vi "Display Dialog.vi"(8 "error in (no error)":errorcluster, 10 "Argument":string, 11 "State Data":T1={"Core"={"Current VI Reference"=refnum, "Close Panel on Exit?"=FALSE}, "FP Refs"={"VI Tree"=refnum, "Window Title"=refnum, "Same Title as VI?"=refnum, "VI Desc"=refnum, "Help Path"=refnum, "Help Tag"=refnum, "Help URL"=refnum, "Help Type"=refnum, "Controls"=refnum, "VI Connector Pane"=refnum, "Path to VI"=refnum, "Inlined?"=refnum, "Allow Debugging?"=refnum, "Auto Error Handling?"=refnum, "Run When Opened?"=refnum, "Suspend When Called?"=refnum, "Reentrancy"=refnum, "Priority"=refnum, "Preferred Exec System"=refnum, "VI Type"=refnum, "Help Properties"=refnum, "Edit Icon"=refnum, "Add Copyright"=refnum, "Set all VIs"=refnum}, "Current Path"=path "", "New Item Data"=[], "Saved Item Data"=[], "FP"={"Selected VI Data"=0, "Help Path"="", "Help Tag"="", "Help URL"="", "Help Type"=enum."Local Help File", "VI Desc"="", "Controls"=[], "Window Title"="", "Same Title?"=FALSE, "VI Tree Value"=""}, "Config Path"=path "", "Config"={"ItemsEdited"=0, "Copyright Path"=path "", "Copyright Delimiter"="", "Recent Folders"=[], "Recent Files"=[], "Recent Filters"=[], "Abbreviate Names?"=FALSE, "Format Bold Tags?"=FALSE, "Show ConPane Only?"=FALSE, "Show Top-Level Only?"=FALSE, "Confirm Save?"=FALSE, "Confirm Revert?"=FALSE, "Confirm Save All?"=FALSE, "Confirm Revert All?"=FALSE, "Confirm Exit?"=FALSE, "Flat View?"=FALSE, "Ctls Sort Column"=0, "Ctls Sort Order"=0}, "Desc Selection"={"Selection Start"=0, "Selection End"=0}, "Displayed Indices"=[], "Filter"={"Filter Column"=enum."Description", "Filter Type"=enum."Contains", "Filter Value"="", "New Data?"=FALSE, "Case Sensitive?"=FALSE, "Enabled?"=FALSE}, "Sort"={"Sort Column"=enum."Description", "Ascending?"=FALSE, "Enabled?"=FALSE}, "Tree Map"=refnum, "Last Save Count"=0, "View Saved?"=FALSE, "Selected Item"=refnum}) -> (0 "error out":errorcluster, 1 "States at Back":string, 2 "States at Front":string, 3 "State Data out":T1={"Core"={"Current VI Reference"=refnum, "Close Panel on Exit?"=FALSE}, "FP Refs"={"VI Tree"=refnum, "Window Title"=refnum, "Same Title as VI?"=refnum, "VI Desc"=refnum, "Help Path"=refnum, "Help Tag"=refnum, "Help URL"=refnum, "Help Type"=refnum, "Controls"=refnum, "VI Connector Pane"=refnum, "Path to VI"=refnum, "Inlined?"=refnum, "Allow Debugging?"=refnum, "Auto Error Handling?"=refnum, "Run When Opened?"=refnum, "Suspend When Called?"=refnum, "Reentrancy"=refnum, "Priority"=refnum, "Preferred Exec System"=refnum, "VI Type"=refnum, "Help Properties"=refnum, "Edit Icon"=refnum, "Add Copyright"=refnum, "Set all VIs"=refnum}, "Current Path"=path "", "New Item Data"=[], "Saved Item Data"=[], "FP"={"Selected VI Data"=0, "Help Path"="", "Help Tag"="", "Help URL"="", "Help Type"=enum."Local Help File", "VI Desc"="", "Controls"=[], "Window Title"="", "Same Title?"=FALSE, "VI Tree Value"=""}, "Config Path"=path "", "Config"={"ItemsEdited"=0, "Copyright Path"=path "", "Copyright Delimiter"="", "Recent Folders"=[], "Recent Files"=[], "Recent Filters"=[], "Abbreviate Names?"=FALSE, "Format Bold Tags?"=FALSE, "Show ConPane Only?"=FALSE, "Show Top-Level Only?"=FALSE, "Confirm Save?"=FALSE, "Confirm Revert?"=FALSE, "Confirm Save All?"=FALSE, "Confirm Revert All?"=FALSE, "Confirm Exit?"=FALSE, "Flat View?"=FALSE, "Ctls Sort Column"=0, "Ctls Sort Order"=0}, "Desc Selection"={"Selection Start"=0, "Selection End"=0}, "Displayed Indices"=[], "Filter"={"Filter Column"=enum."Description", "Filter Type"=enum."Contains", "Filter Value"="", "New Data?"=FALSE, "Case Sensitive?"=FALSE, "Enabled?"=FALSE}, "Sort"={"Sort Column"=enum."Description", "Ascending?"=FALSE, "Enabled?"=FALSE}, "Tree Map"=refnum, "Last Save Count"=0, "View Saved?"=FALSE, "Selected Item"=refnum})   [LabVIEW 2020, in "VI Properties Editor.lvlib"]
doc: "Displays an appropriate dialog according to <B>Argument</B>, and outputs any states that should be enqueued after the dialog is closed."
uses:
  VI Properties Editor.lvlib
  CTLs/Main State Data.ctl
  Classes/Tree Map/Project Tree Map.lvclass
  Classes/Item/Item.lvclass
  CTLs/Main References.ctl
  CTLs/Main Front Panel Controls.ctl
  CTLs/Config.ctl
  CTLs/Filter Info.ctl
  CTLs/Filter Column.ctl
  CTLs/Filter Type.ctl
  <vilib>/Utility/miscctls.llb/LVSelectionTypeDef.ctl
  CTLs/Sort Info.ctl
  CTLs/Sort Column.ctl
  CTLs/Confirmation Type.ctl
  <vilib>/LabVIEW Icon API/lv_icon/Classes/Icon/Icon.lvclass
  <vilib>/LabVIEW Icon API/LabVIEW Icon API.lvlib
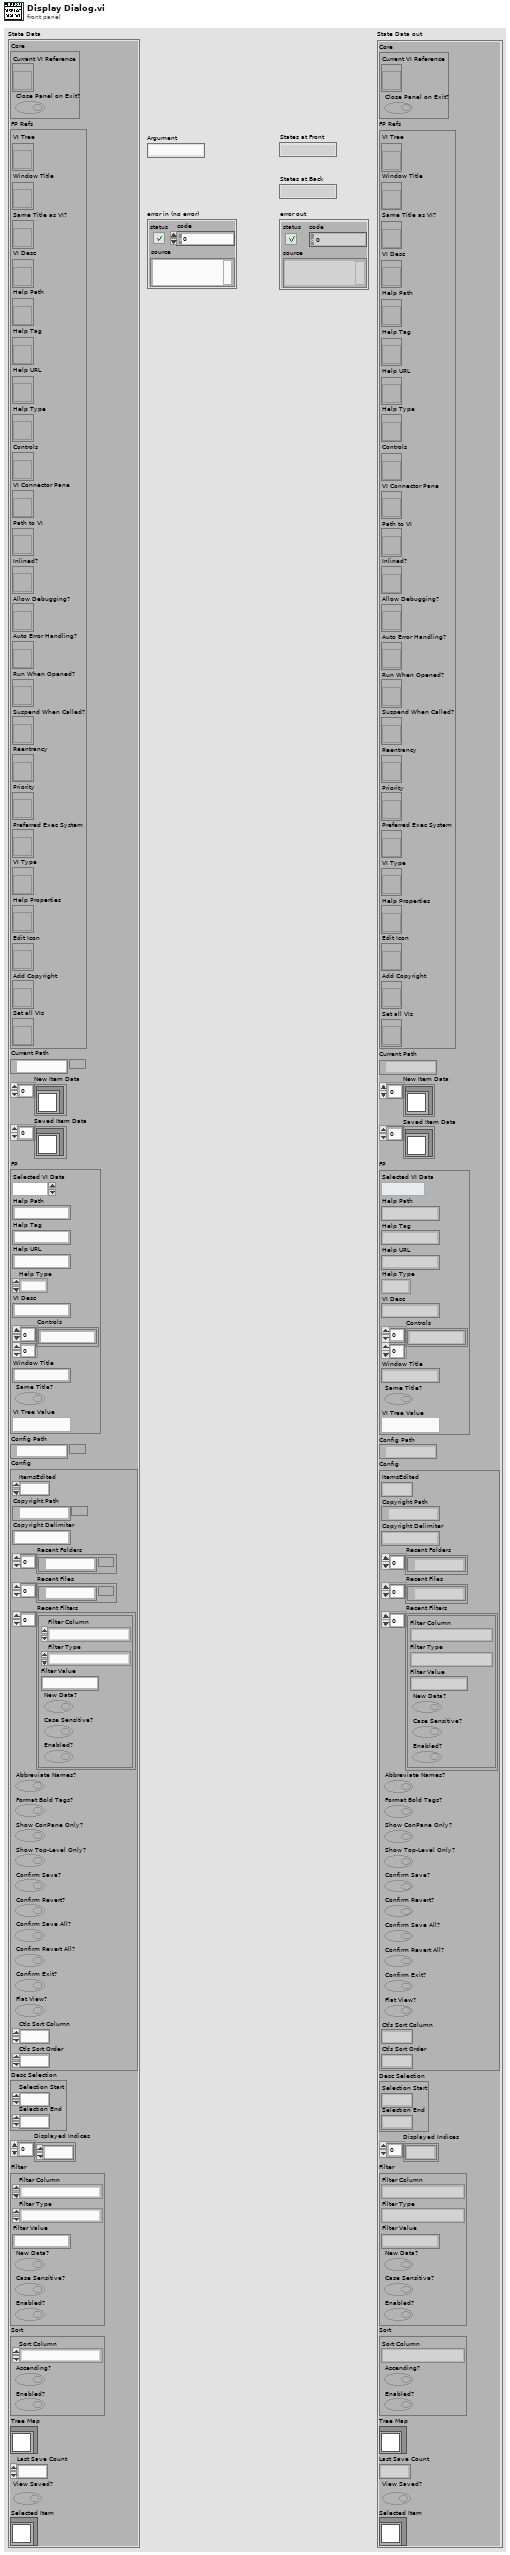
[diagram p1: front panel]
types:
  T1 = typedef "VI Properties Editor.lvlib/Main State Data.ctl" = cluster{"Core":cluster{"Current VI Reference":refnum<vi>, "Close Panel on Exit?":bool}, "FP Refs":T2, "Current Path":path, "New Item Data":refnum<class "Item.lvclass">[], "Saved Item Data":refnum<class "Item.lvclass">[], "FP":T3, "Config Path":path, "Config":T4, "Desc Selection":T8, "Displayed Indices":i32[], "Filter":T5, "Sort":T9, "Tree Map":refnum<class "Project Tree Map.lvclass">, "Last Save Count":u32, "View Saved?":bool, "Selected Item":refnum<class "Item.lvclass">}
  T2 = typedef "VI Properties Editor.lvlib/Main References.ctl" = cluster{"VI Tree":refnum<vi>, "Window Title":refnum<vi>, "Same Title as VI?":refnum<vi>, "VI Desc":refnum<vi>, "Help Path":refnum<vi>, "Help Tag":refnum<vi>, "Help URL":refnum<vi>, "Help Type":refnum<vi>, "Controls":refnum<vi>, "VI Connector Pane":refnum<vi>, "Path to VI":refnum<vi>, "Inlined?":refnum<vi>, "Allow Debugging?":refnum<vi>, "Auto Error Handling?":refnum<vi>, "Run When Opened?":refnum<vi>, "Suspend When Called?":refnum<vi>, "Reentrancy":refnum<vi>, "Priority":refnum<vi>, "Preferred Exec System":refnum<vi>, "VI Type":refnum<vi>, "Help Properties":refnum<vi>, "Edit Icon":refnum<vi>, "Add Copyright":refnum<vi>, "Set all VIs":refnum<vi>}
  T3 = typedef "VI Properties Editor.lvlib/Main Front Panel Controls.ctl" = cluster{"Selected VI Data":i32, "Help Path":string, "Help Tag":string, "Help URL":string, "Help Type":enum16{"Local Help File", "Web-based Help"}, "VI Desc":string, "Controls":string[][], "Window Title":string, "Same Title?":bool, "VI Tree Value":string}
  T4 = typedef "VI Properties Editor.lvlib/Config.ctl" = cluster{"ItemsEdited":u32, "Copyright Path":path, "Copyright Delimiter":string, "Recent Folders":path[], "Recent Files":path[], "Recent Filters":T5[], "Abbreviate Names?":bool, "Format Bold Tags?":bool, "Show ConPane Only?":bool, "Show Top-Level Only?":bool, "Confirm Save?":bool, "Confirm Revert?":bool, "Confirm Save All?":bool, "Confirm Revert All?":bool, "Confirm Exit?":bool, "Flat View?":bool, "Ctls Sort Column":i32, "Ctls Sort Order":i32}
  T5 = typedef "VI Properties Editor.lvlib/Filter Info.ctl" = cluster{"Filter Column":T6, "Filter Type":T7, "Filter Value":string, "New Data?":bool, "Case Sensitive?":bool, "Enabled?":bool}
  T6 = typedef "VI Properties Editor.lvlib/Filter Column.ctl" = enum16{"Name", "Path", "Type", "Window Title", "Description", "Help Path", "Help Tag", "Custom Title?", "Reentrancy", "Inlined?", "Help URL", "Help Type", "Allow Debugging?", "Auto Error Handling?", "Run When Opened?", "Suspend When Called?", "Priority", "Preferred Exec Sytem", "Control Label", "Control Caption", "Control Description", "Control Tip Strip"}
  T7 = typedef "VI Properties Editor.lvlib/Filter Type.ctl" = enum16{"Contains", "Equals", "Starts with", "Ends with", "Is empty", "Does not contain", "Does not equal", "Is not empty"}
  T8 = typedef "LVSelectionTypeDef.ctl" = cluster{"Selection Start":u32, "Selection End":u32}
  T9 = typedef "VI Properties Editor.lvlib/Sort Info.ctl" = cluster{"Sort Column":T10, "Ascending?":bool, "Enabled?":bool}
  T10 = typedef "VI Properties Editor.lvlib/Sort Column.ctl" = enum16{"Name", "Filename", "Path", "Type", "Window Title", "Description", "Help Path", "Help Tag", "Custom Title?", "Reentrancy", "Inlined?", "Help URL", "Help Type", "Allow Debugging?", "Auto Error Handling?", "Run When Opened?", "Suspend When Called?", "Priority", "Preferred Exec Sytem"}
  T11 = enum16{"Left Button", "Center Button", "Right Button", "Window Close"}
  T12 = typedef "VI Properties Editor.lvlib/Confirmation Type.ctl" = enum16{"Save", "Revert", "Save All", "Revert All", "Exit"}
  T13 = typedef "VI Properties Editor.lvlib/Replace Info.ctl" = cluster{"Filter Column":T6, "Filter Type":T7, "Filter Value":string, "Case Sensitive?":bool, "Replace Column":T14, "Replace Value":string}
  T14 = typedef "VI Properties Editor.lvlib/Replace Column.ctl" = enum16{"Window Title", "Description", "Help Path", "Help Tag", "Custom Title?", "Help URL", "Help Type", "Control Label", "Control Caption", "Control Description", "Control Tip Strip"}
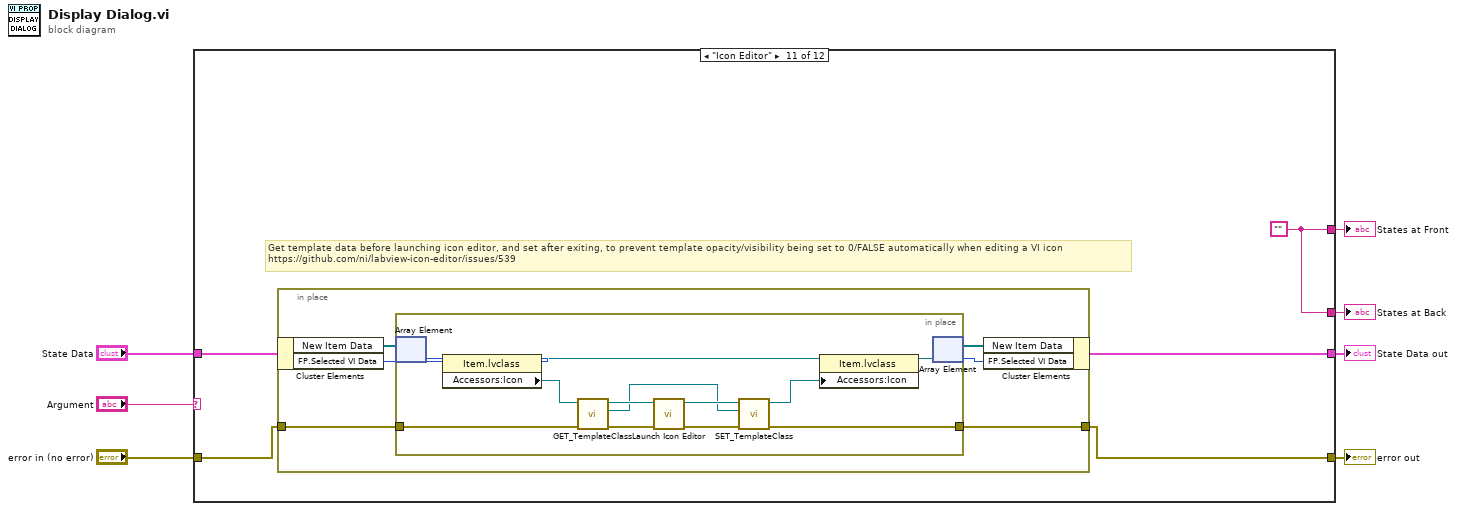
[diagram p0: block diagram]
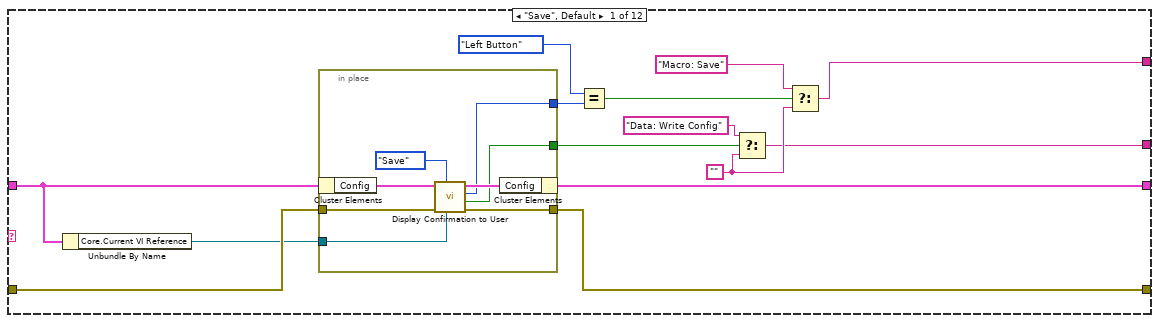
[diagram p2: hidden frame]
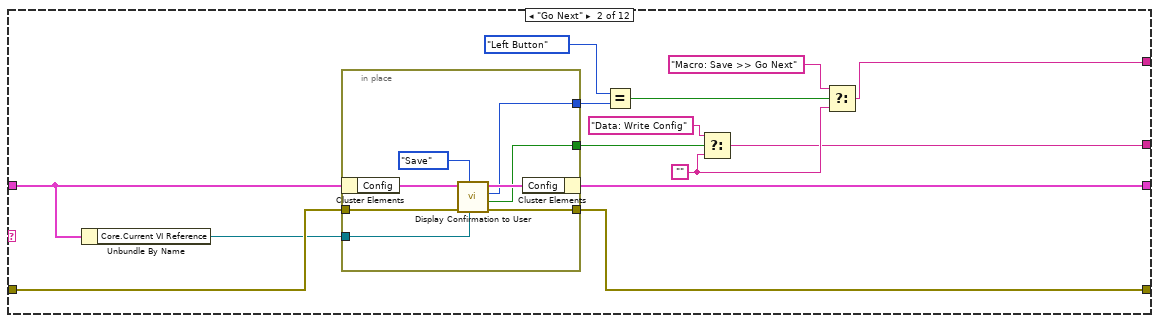
[diagram p3: hidden frame]
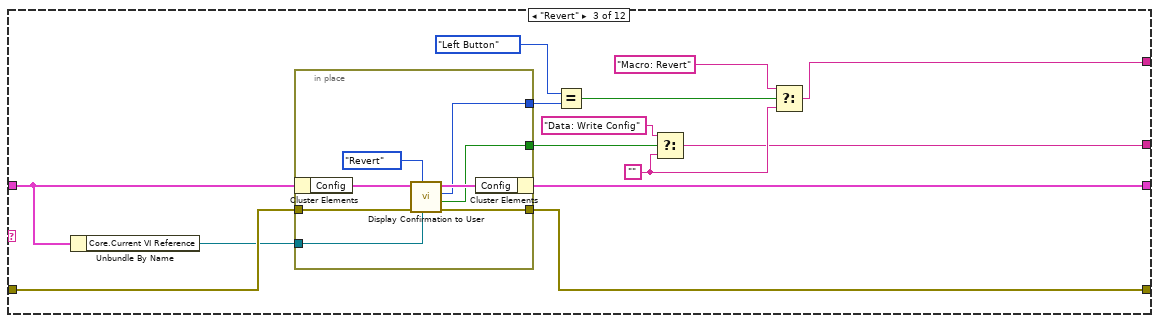
[diagram p4: hidden frame]
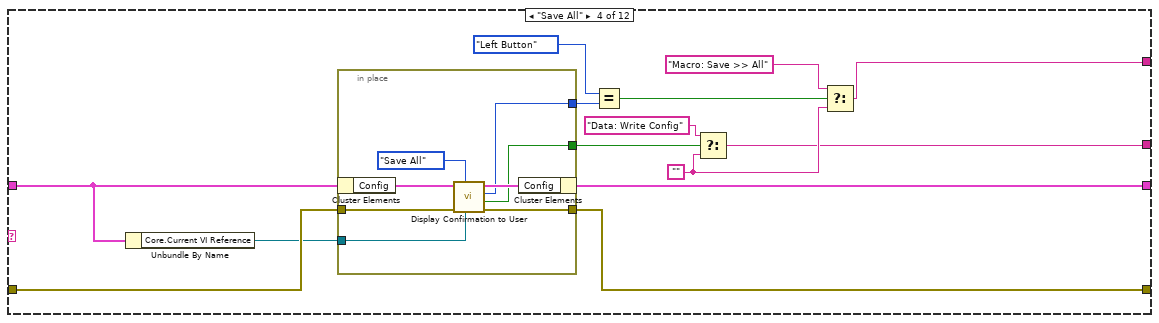
[diagram p5: hidden frame]
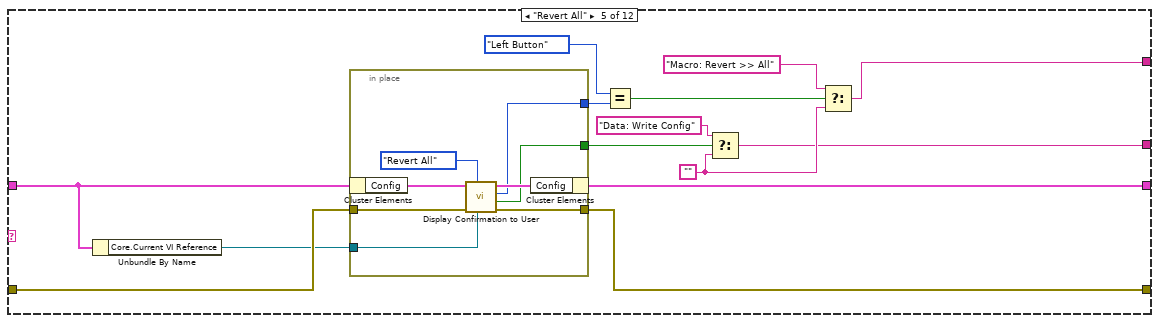
[diagram p6: hidden frame]
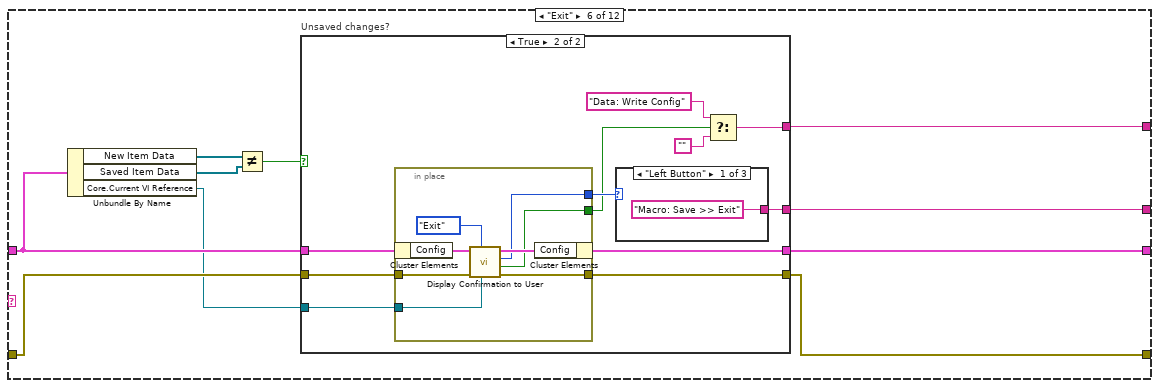
[diagram p7: hidden frame]
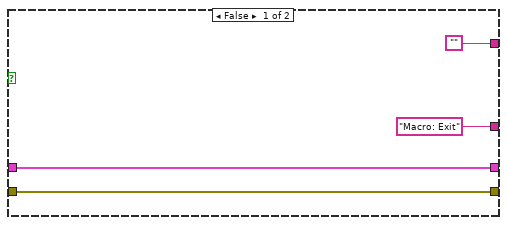
[diagram p8: hidden frame]
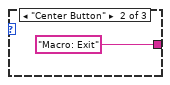
[diagram p9: hidden frame]
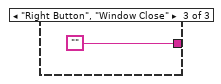
[diagram p10: hidden frame]
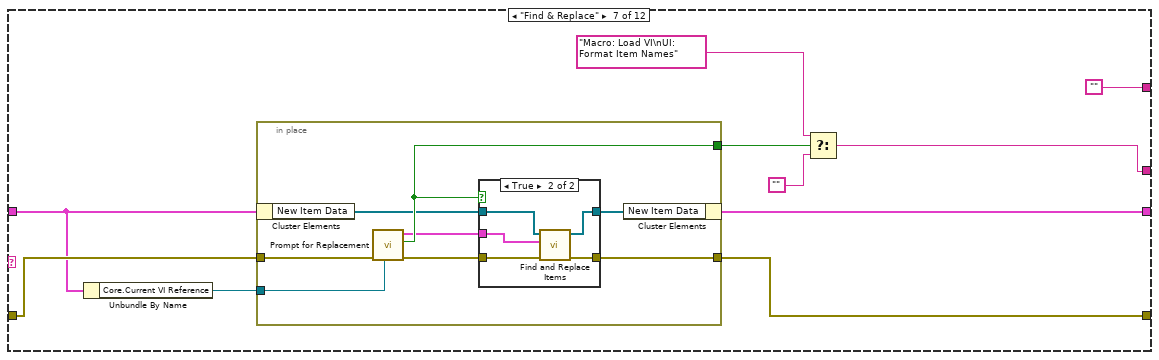
[diagram p11: hidden frame]
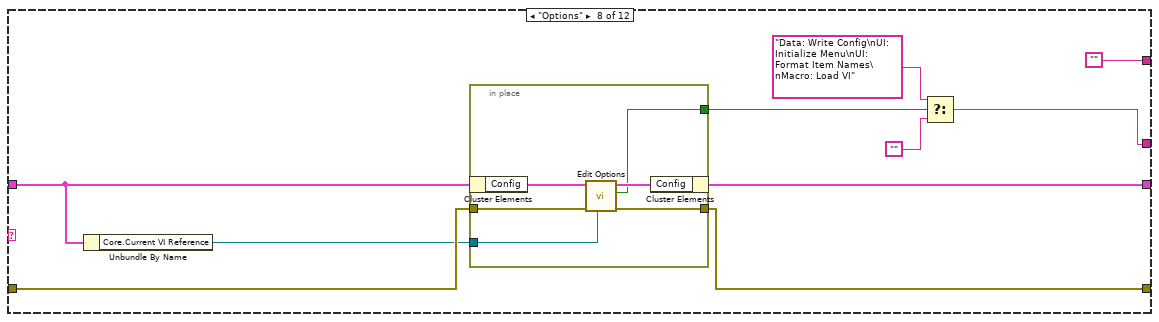
[diagram p13: hidden frame]
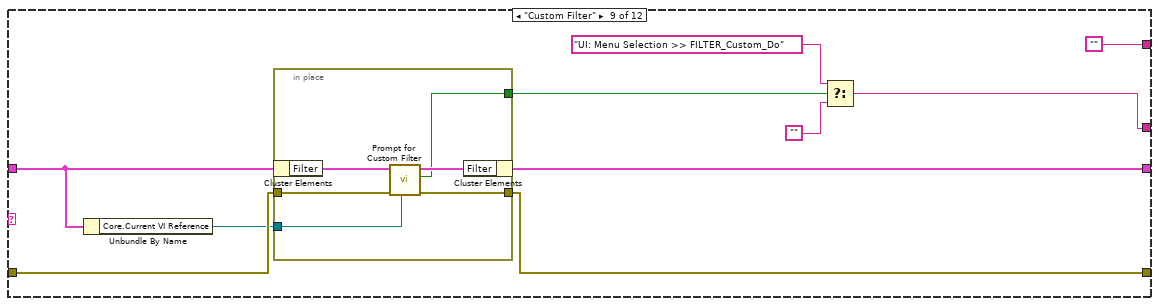
[diagram p14: hidden frame]
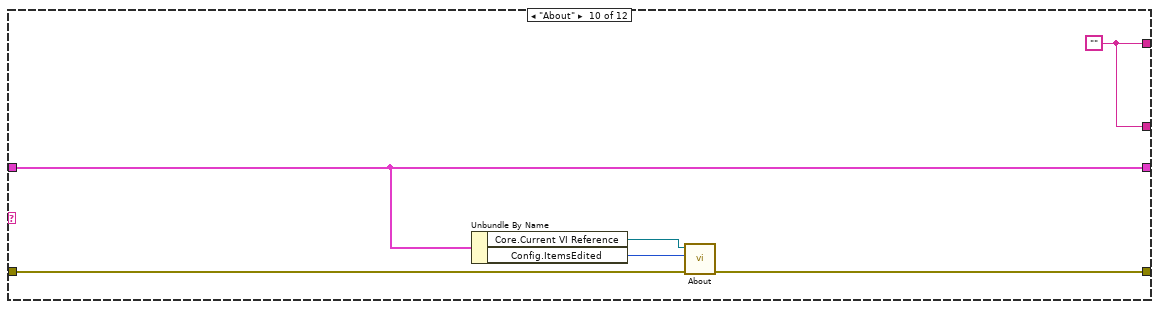
[diagram p15: hidden frame]
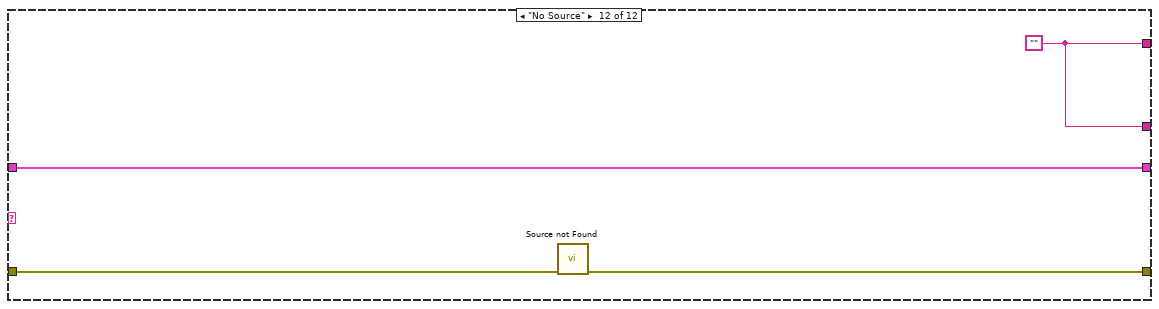
[diagram p16: hidden frame]
diagram:
  n1 = case shown="\"Icon Editor\"" "Argument" {
    tunnel: [w13 w35 w58 w80 w102 w125 "" "" "" w216 w221 w243] -> w2
    tunnel: "error in (no error)" -> [w21 w43 w65 w87 w109 w122 w160 w183 w199 w214 w220 w241]
    tunnel: "State Data" -> [w9 w31 w53 w75 w97 w123 w159 w184 w200 w212 w217 w242]
    tunnel: [w20 w42 w64 w86 w108 w121 w157 w181 w198 w213 w219 w240] -> w4
    tunnel: [w19 w41 w63 w85 w107 w120 w156 w182 w195 w212 w218 w242] -> w6
    tunnel: [w14 w36 w57 w79 w101 w119 w155 w180 w196 w216 w221 w243] -> w3
    frame "Save", Default {
      w16 = ""
      n2 = Unbundle By Name(w9) -> ("Core.Current VI Reference"=w8:refnum<vi>)
      n3 = in-place {
        in-place-border: w21 -> [w28]
        in-place-border: [w26] -> w20
        in-place-border: [w24] -> w18
        in-place-border: [w23] -> w11
        in-place-border: w8 -> [w22]
        n4 = in-place-cluster #1(w9) -> ("Config"=w29:T4)
        n5 = call "Display Confirmation to User.vi"("Calling VI in"=w22, "Confirmation Type"=Confirmation_Type."Save", "error in (no error)"=w28, "Config"=w29) -> ("error out"=w26:errorcluster, "New Config?"=w24:bool, "Which Button?"=w23:T11, "Config out"=w27:T4)  [unwired: 4 in]
        n6 = in-place-cluster #1("Config"=w27) -> (w19:T1)
      }
      n7 = Equal?(x=T11."Left Button", y=w11) -> (x = y?=w10:bool)
      n8 = Select(t="Data: Write Config", s=w18, f=w16) -> (s? t:f=w14:string)
      n9 = Select(t="Macro: Save", s=w10, f=w16) -> (s? t:f=w13:string)
    }
    frame "Go Next" {
      w38 = ""
      n10 = Unbundle By Name(w31) -> ("Core.Current VI Reference"=w30:refnum<vi>)
      n11 = in-place {
        in-place-border: w43 -> [w50]
        in-place-border: [w48] -> w42
        in-place-border: [w46] -> w40
        in-place-border: [w45] -> w33
        in-place-border: w30 -> [w44]
        n12 = in-place-cluster #2(w31) -> ("Config"=w51:T4)
        n13 = call "Display Confirmation to User.vi"("Calling VI in"=w44, "Confirmation Type"=Confirmation_Type."Save", "error in (no error)"=w50, "Config"=w51) -> ("error out"=w48:errorcluster, "New Config?"=w46:bool, "Which Button?"=w45:T11, "Config out"=w49:T4)  [unwired: 4 in]
        n14 = in-place-cluster #2("Config"=w49) -> (w41:T1)
      }
      n15 = Equal?(x=T11."Left Button", y=w33) -> (x = y?=w32:bool)
      n16 = Select(t="Data: Write Config", s=w40, f=w38) -> (s? t:f=w36:string)
      n17 = Select(t="Macro: Save >> Go Next", s=w32, f=w38) -> (s? t:f=w35:string)
    }
    frame "Revert" {
      w60 = ""
      n18 = Unbundle By Name(w53) -> ("Core.Current VI Reference"=w52:refnum<vi>)
      n19 = in-place {
        in-place-border: w65 -> [w72]
        in-place-border: [w70] -> w64
        in-place-border: [w68] -> w62
        in-place-border: [w67] -> w55
        in-place-border: w52 -> [w66]
        n20 = in-place-cluster #3(w53) -> ("Config"=w73:T4)
        n21 = call "Display Confirmation to User.vi"("Calling VI in"=w66, "Confirmation Type"=Confirmation_Type."Revert", "error in (no error)"=w72, "Config"=w73) -> ("error out"=w70:errorcluster, "New Config?"=w68:bool, "Which Button?"=w67:T11, "Config out"=w71:T4)  [unwired: 4 in]
        n22 = in-place-cluster #3("Config"=w71) -> (w63:T1)
      }
      n23 = Equal?(x=T11."Left Button", y=w55) -> (x = y?=w54:bool)
      n24 = Select(t="Data: Write Config", s=w62, f=w60) -> (s? t:f=w57:string)
      n25 = Select(t="Macro: Revert", s=w54, f=w60) -> (s? t:f=w58:string)
    }
    frame "Save All" {
      w82 = ""
      n26 = Unbundle By Name(w75) -> ("Core.Current VI Reference"=w74:refnum<vi>)
      n27 = in-place {
        in-place-border: w87 -> [w94]
        in-place-border: [w92] -> w86
        in-place-border: [w90] -> w84
        in-place-border: [w89] -> w77
        in-place-border: w74 -> [w88]
        n28 = in-place-cluster #4(w75) -> ("Config"=w95:T4)
        n29 = call "Display Confirmation to User.vi"("Calling VI in"=w88, "Confirmation Type"=Confirmation_Type."Save All", "error in (no error)"=w94, "Config"=w95) -> ("error out"=w92:errorcluster, "New Config?"=w90:bool, "Which Button?"=w89:T11, "Config out"=w93:T4)  [unwired: 4 in]
        n30 = in-place-cluster #4("Config"=w93) -> (w85:T1)
      }
      n31 = Equal?(x=T11."Left Button", y=w77) -> (x = y?=w76:bool)
      n32 = Select(t="Data: Write Config", s=w84, f=w82) -> (s? t:f=w79:string)
      n33 = Select(t="Macro: Save >> All", s=w76, f=w82) -> (s? t:f=w80:string)
    }
    frame "Revert All" {
      w104 = ""
      n34 = Unbundle By Name(w97) -> ("Core.Current VI Reference"=w96:refnum<vi>)
      n35 = in-place {
        in-place-border: w109 -> [w116]
        in-place-border: [w114] -> w108
        in-place-border: [w112] -> w106
        in-place-border: [w111] -> w100
        in-place-border: w96 -> [w110]
        n36 = in-place-cluster #5(w97) -> ("Config"=w117:T4)
        n37 = call "Display Confirmation to User.vi"("Calling VI in"=w110, "Confirmation Type"=Confirmation_Type."Revert All", "error in (no error)"=w116, "Config"=w117) -> ("error out"=w114:errorcluster, "New Config?"=w112:bool, "Which Button?"=w111:T11, "Config out"=w115:T4)  [unwired: 4 in]
        n38 = in-place-cluster #5("Config"=w115) -> (w107:T1)
      }
      n39 = Equal?(x=T11."Left Button", y=w100) -> (x = y?=w98:bool)
      n40 = Select(t="Data: Write Config", s=w106, f=w104) -> (s? t:f=w101:string)
      n41 = Select(t="Macro: Revert >> All", s=w98, f=w104) -> (s? t:f=w102:string)
    }
    frame "Exit" {
      n42 = Unbundle By Name(w123) -> ("New Item Data"=w127:refnum<class "Item.lvclass">[], "Saved Item Data"=w126:refnum<class "Item.lvclass">[], "Core.Current VI Reference"=w118:refnum<vi>)
      n43 = Not Equal?(x=w127, y=w126) -> (x != y?=w124:bool)
      n44 = case "Unsaved changes?" shown="True" w124 {
        tunnel: ["" w133] -> w125
        tunnel: w123 -> [w131 w142]
        tunnel: w122 -> [w130 w141]
        tunnel: [w130 w140] -> w121
        tunnel: [w131 w137] -> w120
        tunnel: ["Macro: Exit" w138] -> w119
        tunnel: w118 -> [_ w132]
        frame False {
        }
        frame True {
          n45 = in-place {
            in-place-border: w141 -> [w149]
            in-place-border: [w147] -> w140
            in-place-border: [w145] -> w136
            in-place-border: [w144] -> w139
            in-place-border: w132 -> [w143]
            n46 = in-place-cluster #6(w142) -> ("Config"=w150:T4)
            n47 = call "Display Confirmation to User.vi"("Calling VI in"=w143, "Confirmation Type"=Confirmation_Type."Exit", "error in (no error)"=w149, "Config"=w150) -> ("error out"=w147:errorcluster, "New Config?"=w145:bool, "Which Button?"=w144:T11, "Config out"=w148:T4)  [unwired: 4 in]
            n48 = in-place-cluster #6("Config"=w148) -> (w137:T1)
          }
          n49 = case shown="\"Left Button\"" w139 {
            tunnel: ["Macro: Save >> Exit" "Macro: Exit" ""] -> w138
            frame "Left Button" {
            }
            frame "Center Button" {
            }
            frame "Right Button", "Window Close" {
            }
          }
          n50 = Select(t="Data: Write Config", s=w136, f="") -> (s? t:f=w133:string)
        }
      }
    }
    frame "Find & Replace" {
      n51 = Unbundle By Name(w159) -> ("Core.Current VI Reference"=w158:refnum<vi>)
      n52 = in-place {
        in-place-border: w160 -> [w171]
        in-place-border: [w169] -> w157
        in-place-border: [w168] -> w163
        in-place-border: w158 -> [w164]
        n53 = in-place-cluster #7(w159) -> ("New Item Data"=w166:refnum<class "Item.lvclass">[])
        n54 = call "Prompt for Replacement.vi"("Calling VI in"=w164, "error in (no error)"=w171) -> ("error out"=w170:errorcluster, "OK?"=w168:bool, "Replace Info"=w167:T13)  [unwired: 7 in]
        n55 = case shown="True" w168 {
          tunnel: w170 -> [w173 w178]
          tunnel: [w173 w177] -> w169
          tunnel: w167 -> [_ w176]
          tunnel: w166 -> [w172 w175]
          tunnel: [w172 w174] -> w165
          frame False {
          }
          frame True {
            n56 = call "Find and Replace Items.vi"("error in (no error)"=w178, "Replace Info"=w176, "New Item Data"=w175) -> ("error out"=w177:errorcluster, "New Item Data out"=w174:refnum<class "Item.lvclass">[])  [unwired: 6 in, 1 out]
          }
        }
        n57 = in-place-cluster #7("New Item Data"=w165) -> (w156:T1)
      }
      n58 = Select(t="Macro: Load VI\nUI: Format Item Names", s=w163, f="") -> (s? t:f=w155:string)
    }
    frame "Options" {
      n59 = Unbundle By Name(w184) -> ("Core.Current VI Reference"=w179:refnum<vi>)
      n60 = in-place {
        in-place-border: w183 -> [w194]
        in-place-border: [w193] -> w181
        in-place-border: [w190] -> w187
        in-place-border: w179 -> [w189]
        n61 = in-place-cluster #8(w184) -> ("Config"=w192:T4)
        n62 = call "Edit Options.vi"("Calling VI in"=w189, "error in (no error)"=w194, "Config"=w192) -> ("error out"=w193:errorcluster, "OK?"=w190:bool, "Config out"=w191:T4)  [unwired: 6 in]
        n63 = in-place-cluster #8("Config"=w191) -> (w182:T1)
      }
      n64 = Select(t="Data: Write Config\nUI: Initialize Menu\nUI: Format Item Names\nMacro: Load VI", s=w187, f="") -> (s? t:f=w180:string)
    }
    frame "Custom Filter" {
      n65 = Unbundle By Name(w200) -> ("Core.Current VI Reference"=w197:refnum<vi>)
      n66 = in-place {
        in-place-border: w199 -> [w210]
        in-place-border: [w209] -> w198
        in-place-border: [w206] -> w203
        in-place-border: w197 -> [w205]
        n67 = in-place-cluster #9(w200) -> ("Filter"=w208:T5)
        n68 = call "Prompt for Custom Filter.vi"("Calling VI in"=w205, "error in (no error)"=w210, "Filter Info"=w208) -> ("error out"=w209:errorcluster, "OK?"=w206:bool, "Filter Info out"=w207:T5)  [unwired: 6 in]
        n69 = in-place-cluster #9("Filter"=w207) -> (w195:T1)
      }
      n70 = Select(t="UI: Menu Selection >> FILTER_Custom_Do", s=w203, f="") -> (s? t:f=w196:string)
    }
    frame "About" {
      w216 = ""
      n71 = Unbundle By Name(w212) -> ("Core.Current VI Reference"=w211:refnum<vi>, "Config.ItemsEdited"=w215:u32)
      n72 = call "About.vi"("error in (no error)"=w214, "Items Edited"=w215, "Calling VI in"=w211) -> ("error out"=w213:errorcluster)  [unwired: 8 in]
    }
    frame "Icon Editor" {
      w221 = ""
      # "Get template data before launching icon editor, and set after exiting, to prevent template opacity/visibility being set to 0/FALSE automatically when editing a VI icon\nhttps://github.com/ni/labview-icon-editor/issues/539"
      n73 = in-place {
        in-place-border: w220 -> [w227]
        in-place-border: [w226] -> w219
        n74 = in-place-cluster #10(w217) -> ("New Item Data"=w225:refnum<class "Item.lvclass">[], "FP.Selected VI Data"=w224:i32)
        n75 = in-place {
          in-place-border: w227 -> [w236]
          in-place-border: [w229] -> w226
          n76 = in-place-array #11(w225, w224) -> (w239:refnum<class "Item.lvclass">)
          n77 = property class="Item.lvclass"(reference=w239) -> (reference out=w237:refnum<class "Item.lvclass">, "Accessors:Icon"=w235:refnum<class "Icon.lvclass">)  [unwired: 1 in, 1 out]
          n78 = call-dynamic "GET_TemplateClass.vi"("error in (no error)"=w236, "Icon.lvclass in"=w235) -> ("error out"=w234:errorcluster, "Icon Framework.lvclass"=w230:refnum<class "Icon Framework.lvclass">, "Icon.lvclass out"=w233:refnum<class "Icon.lvclass">)  [unwired: 7 in]
          n79 = call <vilib>:"Launch Icon Editor.vi"("error in (no error)"=w234, "Icon in"=w233) -> ("error out"=w232:errorcluster, "Icon out"=w231:refnum<class "Icon.lvclass">)  [unwired: 7 in, 1 out]
          n80 = call-dynamic "SET_TemplateClass.vi"("error in (no error)"=w232, "Icon Framework.lvclass"=w230, "Icon.lvclass in"=w231) -> ("error out"=w229:errorcluster, "Icon.lvclass out"=w228:refnum<class "Icon.lvclass">)  [unwired: 7 in]
          n81 = property class="Item.lvclass"(reference=w237, "Accessors:Icon"=w228) -> (reference out=w238:refnum<class "Item.lvclass">)  [unwired: 1 in, 1 out]
          n82 = in-place-array #11(w238) -> (w223:refnum<class "Item.lvclass">[], w222:i32)
        }
        n83 = in-place-cluster #10("New Item Data"=w223, "FP.Selected VI Data"=w222) -> (w218:T1)
      }
    }
    frame "No Source" {
      w243 = ""
      n84 = call "Source not Found"("error in (no error)"=w241) -> ("error out"=w240:errorcluster)  [unwired: 9 in, 1 out]
    }
  }
  "State Data out" <- w6
  "error out" <- w4
  "States at Back" <- w3
  "States at Front" <- w2
